vi "Find Regulation Target Crossing.vi"(8 "error in (no error)":errorcluster, 10 "sweep start frequency (Hz)":dbl, 11 "measurement configuration":T1 {"acq sampling rate" format="%0.2f"; "master clock rate" format="%#_6pHz"; "frame clock rate" format="%#_6pHz"}) -> (0 "error out":errorcluster, 1 "search results":cluster{"level":dbl, "value":dbl}[](array[cluster]), 2 "crossing found?":bool, 3 "measurement configuration out":T1={"digital channel list"="7821\\PCMo 8", "frame clock rate"=48000.0, "number of channels"=2, "channel length"=32, "bit depth"=24, "data justification"=enum."Left Justified", "endianness"=enum."MSB First", "bit clock edge sync"=enum."Falling", "frame sync edge for channel 0"=enum."Falling", "channel 0 offset"=1, "master clock channel list"="7821\\PCMo 0", "master clock rate"=12288000.0, "enable dither"=TRUE, "logic level"=enum."3.3 V", "output level"=-1.0, "output level units"=enum."dBFS", "output range (pk-pk)"=15.0, "load impedance"=4.0, "signal phase"=0.0, "acq sampling rate"=51200.0, "min measurement cycles"=20, "min measurement time (s)"=0.1, "min settling cycles"=0, "min settling time (s)"=0.0, "acq channel"="", "band start"=20.0, "band stop"=20000.0, "weighting filter"=enum."A-weighting", "highpass filter"=enum."DC", "lowpass filter"=enum."No filter", "sweep start frequency (Hz)"=20.0, "sweep stop frequency (Hz)"=20000.0, "number of steps"=10, "sweep profile"=enum."Logarithmic", "SNR units"=enum."dB", "THD+N units"=enum."dB", "THD units"=enum."dB", "gain units"=enum."dB", "enable regulation"=FALSE, "regulation target"=enum."THD+N Level", "regulation target value"=20.0, "regulation target value units"=enum."x/y", "regulation start level"=20.0, "regulation stop level"=20000.0, "regulation number of steps"=20000} {"acq sampling rate" format="%0.2f"; "master clock rate" format="%#_6pHz"; "frame clock rate" format="%#_6pHz"})   [LabVIEW 2021, in "Stepped Frequency Sweep_Class D Amplifier.lvlib"]
uses:
  Stepped Frequency Sweep_Class D Amplifier.lvlib
  Measurement Configuration.ctl
  shared/controls/digital audio protocol/data justification.ctl
  shared/controls/digital audio protocol/endianness.ctl
  shared/controls/digital audio protocol/digital edge.ctl
  shared/controls/digital audio protocol/logic level.ctl
  shared/controls/digital output level units.ctl
  shared/controls/weighting filter.ctl
  shared/controls/highpass filter.ctl
  shared/controls/lowpass filter.ctl
  shared/controls/sweep profile.ctl
  shared/controls/units - snr.ctl
  shared/controls/units - ratio.ctl
  shared/controls/regulation target.ctl
  shared/controls/regulation target value units.ctl
  shared/controls/audio controls.lvlib
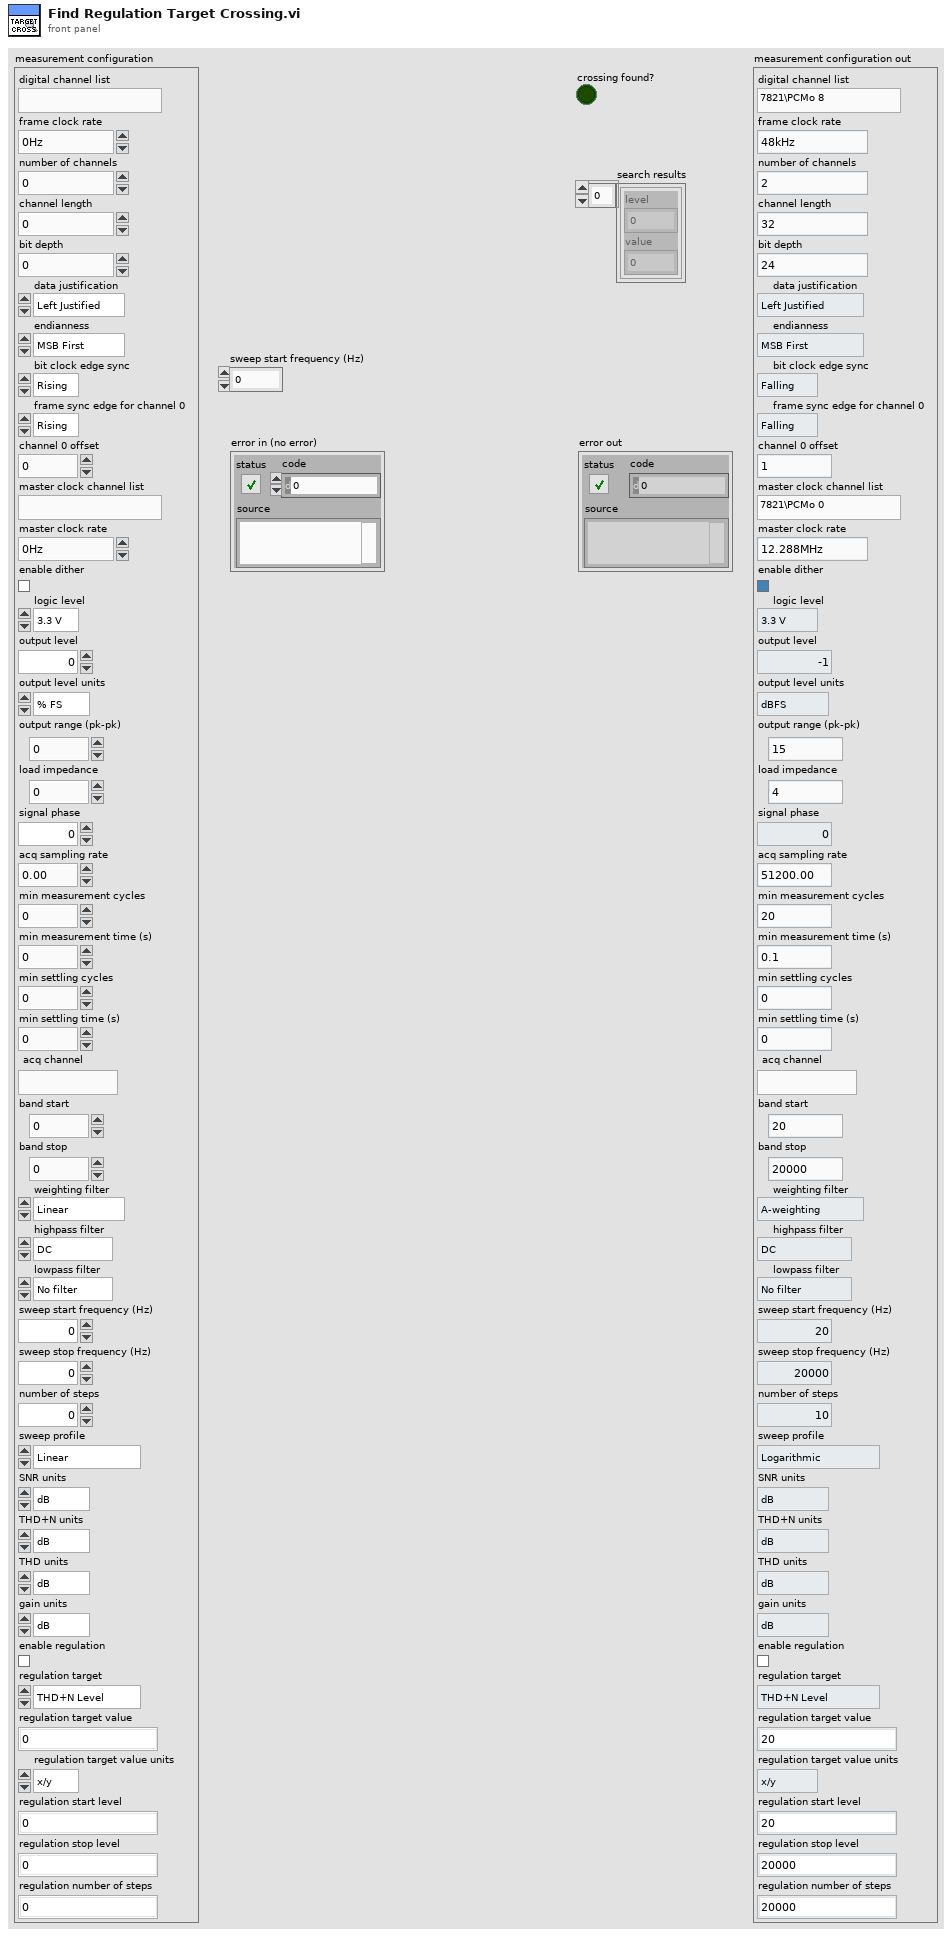
[diagram p1: front panel]
types:
  T1 = typedef "Stepped Frequency Sweep_Class D Amplifier.lvlib/Measurement Configuration.ctl" = cluster{"digital channel list":string, "frame clock rate":dbl, "number of channels":u32, "channel length":u32, "bit depth":u32, "data justification":T2, "endianness":T3, "bit clock edge sync":T4, "frame sync edge for channel 0":T4, "channel 0 offset":u32, "master clock channel list":string, "master clock rate":dbl, "enable dither":bool, "logic level":T5, "output level":dbl, "output level units":T6, "output range (pk-pk)":dbl, "load impedance":dbl, "signal phase":dbl, "acq sampling rate":dbl, "min measurement cycles":u32, "min measurement time (s)":dbl, "min settling cycles":u32, "min settling time (s)":dbl, "acq channel":string, "band start":dbl, "band stop":dbl, "weighting filter":T7, "highpass filter":T8, "lowpass filter":T9, "sweep start frequency (Hz)":dbl, "sweep stop frequency (Hz)":dbl, "number of steps":u32, "sweep profile":T10, "SNR units":T11, "THD+N units":T12, "THD units":T12, "gain units":T12, "enable regulation":bool, "regulation target":T13, "regulation target value":dbl, "regulation target value units":T14, "regulation start level":dbl, "regulation stop level":dbl, "regulation number of steps":u32}
  T2 = typedef "data justification.ctl" = enum32{"Left Justified", "Right Justified"}
  T3 = typedef "endianness.ctl" = enum32{"MSB First", "LSB First"}
  T4 = typedef "digital edge.ctl" = enum32{"Rising", "Falling"}
  T5 = typedef "logic level.ctl" = enum32{"3.3 V", "1.8 V", "1.2 V"}
  T6 = typedef "audio controls.lvlib/digital output level units.ctl" = enum32{"% FS", "dBFS"}
  T7 = typedef "weighting filter.ctl" = enum32{"Linear", "A-weighting", "B-weighting", "C-weighting"}
  T8 = typedef "highpass filter.ctl" = enum32{"DC", "AC"}
  T9 = typedef "lowpass filter.ctl" = enum32{"No filter", "AES17 20kHz", "AES17 40kHz"}
  T10 = typedef "audio controls.lvlib/sweep profile.ctl" = enum32{"Linear", "Logarithmic"}
  T11 = typedef "audio controls.lvlib/units - snr.ctl" = enum32{"dB", "x/y"}
  T12 = typedef "audio controls.lvlib/units - ratio.ctl" = enum32{"dB", "%", "x/y"}
  T13 = typedef "regulation target.ctl" = enum32{"THD+N Level", "THD+N Ratio", "RMS Level", "RMS Ratio", "Output Power"}
  T14 = typedef "regulation target value units.ctl" = enum32{"x/y", "%", "dB", "Vrms", "W"}
  T15 = typedef "audio controls.lvlib/single tone audio measurements.ctl" = cluster{"channel":string, "frequency (Hz)":dbl, "amplitude (Vrms)":dbl, "amplitude (dBFS)":dbl, "phase (deg)":dbl, "SNR":dbl, "THD+N":dbl, "THD":dbl, "dynamic range (dB)":dbl, "gain":dbl, "SFDR (dBc)":dbl}
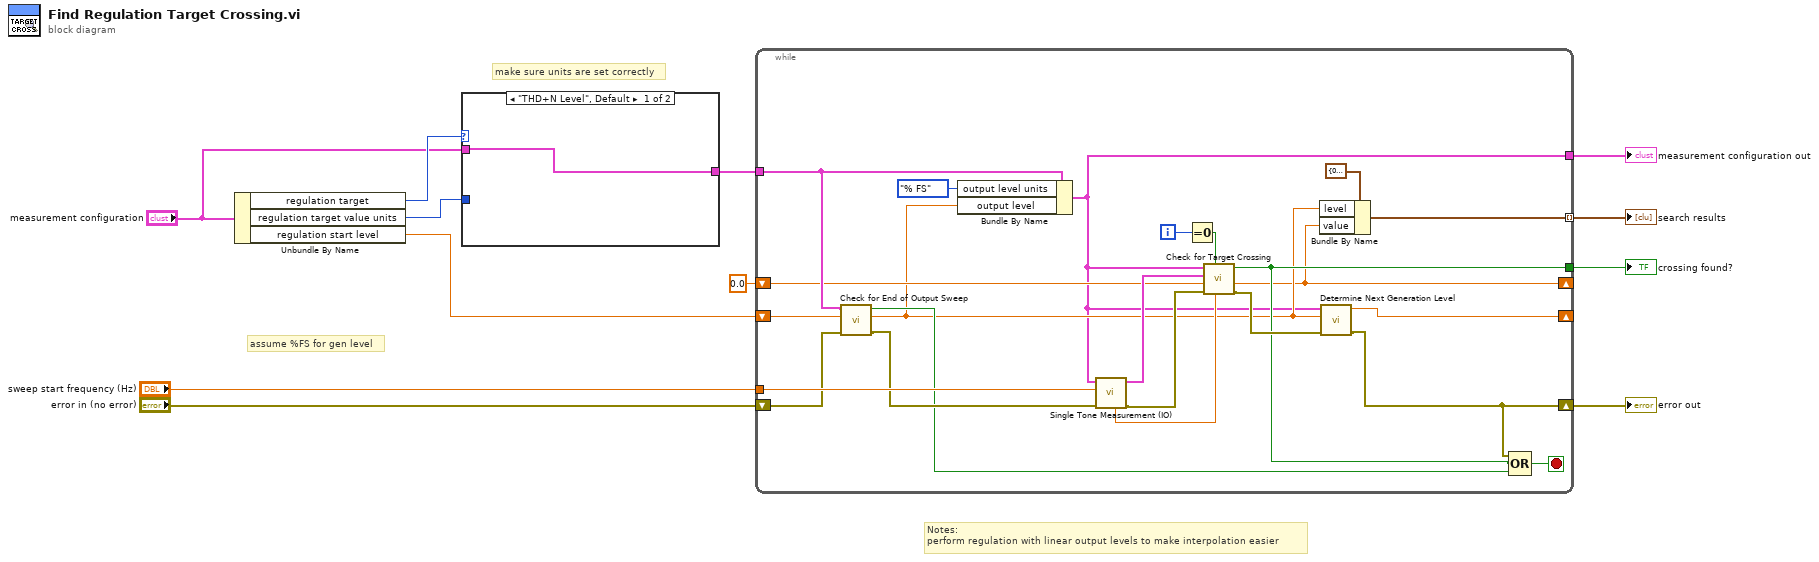
[diagram p0: block diagram]
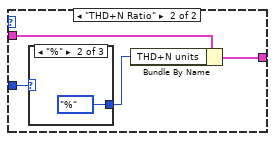
[diagram p2: hidden frame]
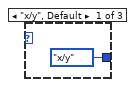
[diagram p3: hidden frame]
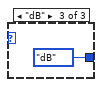
[diagram p4: hidden frame]
diagram:
  # "make sure units are set correctly"
  # "assume %FS for gen level"
  # "Notes:\nperform regulation with linear output levels to make interpolation easier"
  n1 = Unbundle By Name("measurement configuration") -> ("regulation target"=w7:T13, "regulation target value units"=w5:T14, "regulation start level"=w9:dbl)
  n2 = case shown="\"THD+N Level\", Default" w7 {
    tunnel: [w13 w17] -> w8
    tunnel: "measurement configuration" -> [w13 w15]
    tunnel: w5 -> [_ w14]
    frame "THD+N Level", Default {
    }
    frame "THD+N Ratio" {
      n3 = case shown="\"%\"" w14 {
        tunnel: [units_-_ratio."x/y" ("THD+N units") units_-_ratio."%" ("THD+N units") units_-_ratio."dB" ("THD+N units")] -> w16
        frame "x/y", Default {
        }
        frame "%" {
        }
        frame "dB" {
        }
      }
      n4 = Bundle By Name(cluster=w15, "THD+N units"=w16) -> (w17:T1)
    }
  }
  n5 = while {
    shift-right: [w30] -> w11
    shift-left: "error in (no error)" -> [w33]
    tunnel: "sweep start frequency (Hz)" -> [w43]
    shift-right: [w35] -> _
    shift-left: w9 -> [w34]
    tunnel: w8 -> [w31]
    shift-right: [w23] -> _
    shift-left: 0.0 ("measured value") -> [w26]
    tunnel: [w27] -> w3
    tunnel: [w22] -> w2 mode=indexing
    tunnel: [w21] -> w1
    i -> [w38]
    stop <- w28 stop-if-true
    n6 = call "Check for End of Output Sweep.vi"("error in (no error)"=w33, "current generation level"=w34, "measurement configuration"=w31) -> ("error out"=w32:errorcluster, "generation level"=w24:dbl, "sweep done"=w29:bool)  [unwired: 6 in]
    n7 = Bundle By Name(cluster=w31, "output level units"=digital_output_level_units."% FS", "output level"=w24) -> (w21:T1)
    n8 = call "Single Tone Measurement (IO).vi"("error in (no error)"=w32, "sweep start frequency (Hz)"=w43, "measurement configuration"=w21) -> ("error out"=w41:errorcluster, "results"=w39:T15, "output power"=w40:dbl)  [unwired: 4 in, 2 out]
    n9 = Equal To 0?(x=w38) -> (x = 0?=w37:bool)
    n10 = call "Check for Target Crossing.vi"("output power"=w40, "first call?"=w37, "error in (no error)"=w41, "previous measured value"=w26, "results"=w39, "measurement configuration"=w21) -> ("error out"=w36:errorcluster, "measured value"=w23:dbl, "crossing found?"=w27:bool)  [unwired: 3 in]
    n11 = Bundle By Name(cluster=cluster{"level":dbl, "value":dbl} {"level"=0.0, "value"=0.0}, "level"=w24, "value"=w23) -> (w22:cluster{"level":dbl, "value":dbl})
    n12 = call "Determine Next Generation Level.vi"("error in (no error)"=w36, "current generation level"=w24, "measurement configuration"=w21) -> ("error out"=w30:errorcluster, "next generation level"=w35:dbl)  [unwired: 7 in]
    n13 = Compound Arithmetic op=OR(w30, w27, w29) -> (w28:bool)
  }
  "error out" <- w11
  "crossing found?" <- w3
  "search results" <- w2
  "measurement configuration out" <- w1
